vi "Read Controls from Config File.vi"(6 "Child?":bool, 7 "section":string, 8 "Error In":errorcluster, 9 "ParentName":string, 10 "Ctl Refnum":refnum<vi>, 11 "refnum":T1) -> (0 "Error Out":errorcluster, 3 "refnum out":T1)   [LabVIEW 2014]
uses:
  <vilib>/Utility/config.llb/Config Data RefNum.ctl
  Hardware/Table Stage/Controls/Translation Stage Cluster.ctl
  Controls/Translation Stage Types.ctl
  <vilib>/Utility/config.llb/Read Key (String).vi
  <vilib>/Utility/config.llb/Read Key (Boolean).vi
  <vilib>/Utility/config.llb/Read Key (Double).vi
  <vilib>/Utility/config.llb/Read Key (U32).vi
  <vilib>/Utility/config.llb/NI_LVConfig.lvlib
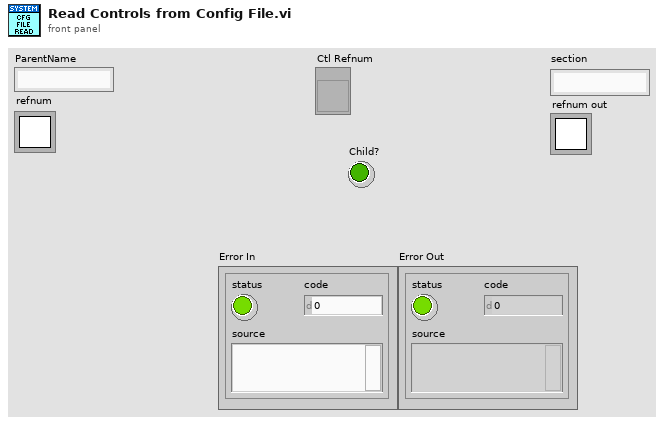
[diagram p1: front panel]
types:
  T1 = typedef "NI_LVConfig.lvlib/Config Data RefNum.ctl" = refnum<k1>
  T2 = typedef "Translation Stage Cluster.ctl" = cluster{"Position":dbl, "Is.Enabled?":bool, "Is.Connected?":bool, "Device SN":string, "AccelerationMaximum":dbl, "VelocityMaximum":dbl, "Acceleration":dbl, "Velocity":dbl, "waitTimeout (ms)":i32, "Model":T3, "Is.Homed?":bool}
  T3 = typedef "Translation Stage Types.ctl" = enum16{"None", "Thorlabs LTS", "Thorlabs MLJ"}
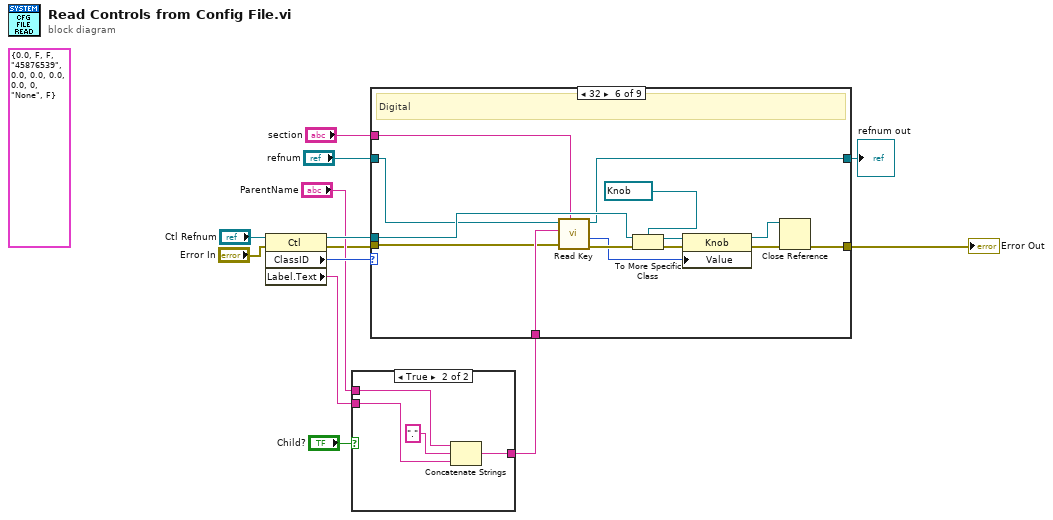
[diagram p0: block diagram]
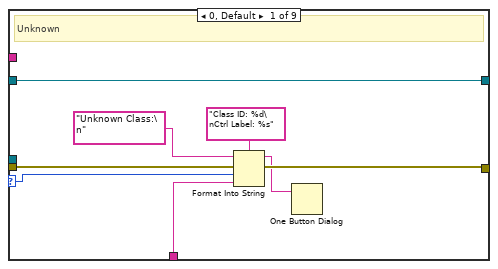
[diagram p3: hidden frame]
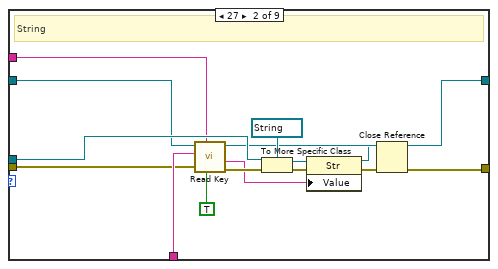
[diagram p4: hidden frame]
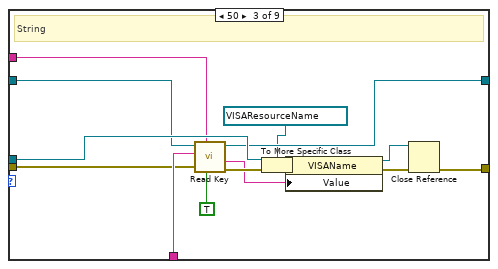
[diagram p5: hidden frame]
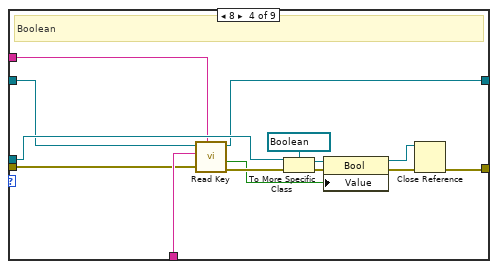
[diagram p6: hidden frame]
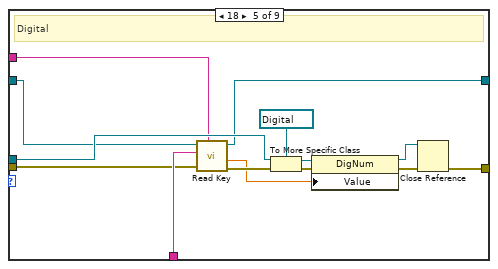
[diagram p7: hidden frame]
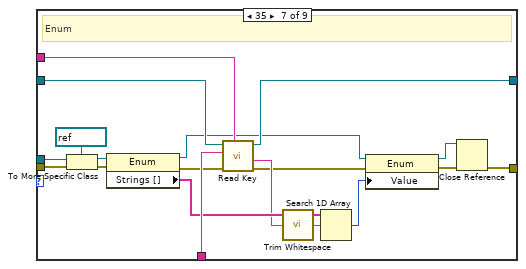
[diagram p8: hidden frame]
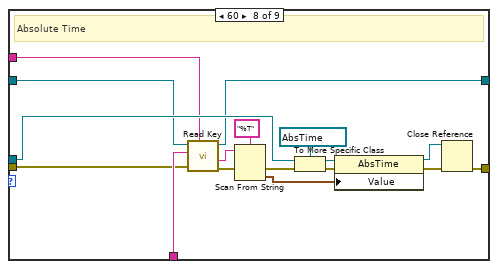
[diagram p9: hidden frame]
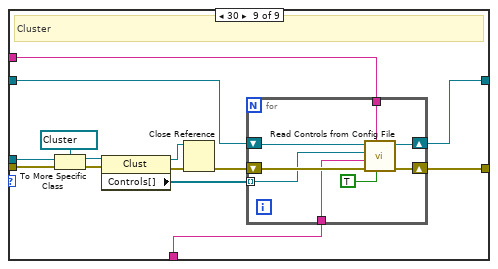
[diagram p10: hidden frame]
diagram:
  (unwired) T2 {"Position"=0.0, "Is.Enabled?"=FALSE, "Is.Connected?"=FALSE, "Device SN"="45876539", "AccelerationMaximum"=0.0, "VelocityMaximum"=0.0, "Acceleration"=0.0, "Velocity"=0.0, "waitTimeout (ms)"=0, "Model"=enum."None", "Is.Homed?"=FALSE} ("Control Param In")
  n1 = property class="Ctl"(reference="Ctl Refnum", error in="Error In") -> (reference out=w12:refnum<vi>, error out=w6:errorcluster, "ClassID"=w11:u32, "Label.Text"=w8:string)
  n2 = case shown="True" "Child?" {
    tunnel: "ParentName" -> [_ w18]
    tunnel: w8 -> [w14 w16]
    tunnel: [w14 w15] -> w3
    frame False {
    }
    frame True {
      n3 = Concatenate Strings(w18, ".", w16) -> (w15:string)
    }
  }
  n4 = case shown="32" w11 {
    selector: w11 -> [w23 _ _ _ _ _ _ _ _]
    tunnel: w6 -> [w21 w30 w46 w58 w72 w87 w116 w122 w147]
    tunnel: w12 -> [_ w40 w56 w68 w83 w97 w115 w133 w145]
    tunnel: [w20 w28 w44 w67 w73 w88 w99 w123 w141] -> w1
    tunnel: "section" -> [_ w39 w55 w66 w76 w91 w111 w127 w138]
    tunnel: "refnum" -> [w26 w38 w54 w65 w75 w90 w110 w126 w140]
    tunnel: [w26 w37 w53 w64 w74 w89 w109 w125 w139] -> w2
    tunnel: w3 -> [w22 w35 w51 w62 w77 w92 w112 w128 w137]
    frame 0, Default {
      # "Unknown"
      n5 = Format Into String(format string="Class ID: %d\nCtrl Label: %s", initial string="Unknown Class:\n" ("string"), error in=w21, w23, w22) -> (resulting string=w19:string, error out=w20:errorcluster)
      n6 = One Button Dialog(message=w19) -> ()  [unwired: 1 in, 1 out]
    }
    frame 27 {
      # "String"
      n7 = call-poly <vilib>:"Read Key.vi"("read raw string? (F)"=TRUE, "section"=w39, "error in (no error)"=w30, "key"=w35, "refnum"=w38) -> ("error out"=w29:errorcluster, "value"=w27:string, "refnum out"=w37:T1)  [unwired: 3 in, 1 out]
      n8 = To More Specific Class(target class=refnum<vi> refnum ("AccelerationMaximum 2"), reference=w40, error in=w29) -> (specific class reference=w33:refnum<vi>, error out=w36:errorcluster)
      n9 = property class="Str"(reference=w33, error in=w36, "Value"=w27) -> (reference out=w32:refnum<vi>, error out=w34:errorcluster)
      n10 = Close Reference(reference=w32, error in (no error)=w34) -> (error out=w28:errorcluster)
    }
    frame 50 {
      # "String"
      n11 = call-poly <vilib>:"Read Key.vi"("read raw string? (F)"=TRUE, "section"=w55, "error in (no error)"=w46, "key"=w51, "refnum"=w54) -> ("error out"=w45:errorcluster, "value"=w43:string, "refnum out"=w53:T1)  [unwired: 3 in, 1 out]
      n12 = To More Specific Class(target class=refnum<vi> refnum ("Controller VISA Ref"), reference=w56, error in=w45) -> (specific class reference=w49:refnum<vi>, error out=w52:errorcluster)
      n13 = property class="VISAName"(reference=w49, error in=w52, "Value"=w43) -> (reference out=w48:refnum<vi>, error out=w50:errorcluster)
      n14 = Close Reference(reference=w48, error in (no error)=w50) -> (error out=w44:errorcluster)
    }
    frame 8 {
      # "Boolean"
      n15 = call-poly <vilib>:"Read Key.vi"("section"=w66, "error in (no error)"=w58, "key"=w62, "refnum"=w65) -> ("error out"=w67:errorcluster, "value"=w57:bool, "refnum out"=w64:T1)  [unwired: 4 in, 1 out]
      n16 = To More Specific Class(target class=refnum<vi> refnum ("AccelerationMaximum 2"), reference=w68) -> (specific class reference=w60:refnum<vi>, error out=w63:errorcluster)  [unwired: 1 in]
      n17 = property class="Bool"(reference=w60, error in=w63, "Value"=w57) -> (reference out=w59:refnum<vi>, error out=w61:errorcluster)
      n18 = Close Reference(reference=w59, error in (no error)=w61) -> ()  [unwired: 1 out]
    }
    frame 18 {
      # "Digital"
      n19 = call-poly <vilib>:"Read Key.vi"("section"=w76, "error in (no error)"=w72, "key"=w77, "refnum"=w75) -> ("error out"=w71:errorcluster, "value"=w70:dbl, "refnum out"=w74:T1)  [unwired: 4 in, 1 out]
      n20 = To More Specific Class(target class=refnum<vi> refnum ("AccelerationMaximum 2"), reference=w83, error in=w71) -> (specific class reference=w80:refnum<vi>, error out=w81:errorcluster)
      n21 = property class="DigNum"(reference=w80, error in=w81, "Value"=w70) -> (reference out=w78:refnum<vi>, error out=w79:errorcluster)
      n22 = Close Reference(reference=w78, error in (no error)=w79) -> (error out=w73:errorcluster)
    }
    frame 32 {
      # "Digital"
      n23 = call-poly <vilib>:"Read Key.vi"("section"=w91, "error in (no error)"=w87, "key"=w92, "refnum"=w90) -> ("error out"=w86:errorcluster, "value"=w85:u32, "refnum out"=w89:T1)  [unwired: 4 in, 1 out]
      n24 = To More Specific Class(target class=refnum<vi> refnum ("Zoom Factor"), reference=w97, error in=w86) -> (specific class reference=w95:refnum<vi>, error out=w96:errorcluster)
      n25 = property class="Knob"(reference=w95, error in=w96, "Value"=w85) -> (reference out=w93:refnum<vi>, error out=w94:errorcluster)
      n26 = Close Reference(reference=w93, error in (no error)=w94) -> (error out=w88:errorcluster)
    }
    frame 35 {
      # "Enum"
      n27 = To More Specific Class(target class=refnum<vi> refnum ("Enum"), reference=w115, error in=w116) -> (specific class reference=w113:refnum<vi>, error out=w114:errorcluster)
      n28 = property class="Enum"(reference=w113, error in=w114) -> (reference out=w100:refnum<vi>, error out=w106:errorcluster, "Strings []"=w107:string[])
      n29 = call-poly <vilib>:"Read Key.vi"("section"=w111, "error in (no error)"=w106, "key"=w112, "refnum"=w110) -> ("error out"=w104:errorcluster, "value"=w105:string, "refnum out"=w109:T1)  [unwired: 4 in, 1 out]
      n30 = call <vilib>:"Trim Whitespace.vi"("string"=w105) -> ("trimmed string"=w102:string)  [unwired: 1 in]
      n31 = Search 1D Array(1D array=w107, element=w102) -> (index of element=w101:i32)  [unwired: 1 in]
      n32 = property class="Enum"(reference=w100, error in=w104, "Value"=w101) -> (reference out=w98:refnum<vi>, error out=w103:errorcluster)
      n33 = Close Reference(reference=w98, error in (no error)=w103) -> (error out=w99:errorcluster)
    }
    frame 60 {
      # "Absolute Time"
      n34 = call-poly <vilib>:"Read Key.vi"("section"=w127, "error in (no error)"=w122, "key"=w128, "refnum"=w126) -> ("error out"=w120:errorcluster, "value"=w117:string, "refnum out"=w125:T1)  [unwired: 4 in, 1 out]
      n35 = Scan From String(format string="%T", input string=w117, error in=w120) -> (error out=w119:errorcluster, output 1=w118:timestamp)  [unwired: 2 in, 2 out]
      n36 = To More Specific Class(target class=refnum<vi> refnum ("AccelerationMaximum 2"), reference=w133, error in=w119) -> (specific class reference=w131:refnum<vi>, error out=w132:errorcluster)
      n37 = property class="AbsTime"(reference=w131, error in=w132, "Value"=w118) -> (reference out=w129:refnum<vi>, error out=w130:errorcluster)
      n38 = Close Reference(reference=w129, error in (no error)=w130) -> (error out=w123:errorcluster)
    }
    frame 30 {
      # "Cluster"
      n39 = To More Specific Class(target class=refnum<vi> refnum ("Cluster Ref In"), reference=w145, error in=w147) -> (specific class reference=w143:refnum<vi>, error out=w144:errorcluster)
      n40 = property class="Clust"(reference=w143, error in=w144) -> (reference out=w135:refnum<vi>, error out=w142:errorcluster, "Controls[]"=w134:refnum<vi>[])
      n41 = Close Reference(reference=w135, error in (no error)=w142) -> (error out=w136:errorcluster)
      n42 = for {
        tunnel: w138 -> [w151]
        tunnel: w137 -> [w150]
        shift-right: [w154] -> w141
        shift-left: w136 -> [w155]
        shift-right: [w152] -> w139
        shift-left: w140 -> [w153]
        tunnel: w134 -> [w148] mode=indexing
        n43 = call "Read Controls from Config File.vi"("Child?"=TRUE, "section"=w151, "Error In"=w155, "ParentName"=w150, "Ctl Refnum"=w148, "refnum"=w153) -> ("Error Out"=w154:errorcluster, "refnum out"=w152:T1)  [unwired: 4 in]
      }
    }
  }
  "Error Out" <- w1
  "refnum out" <- w2
